vi "Self Event Alias.vi"(11 "Base Event in":refnum<class "Base Event.lvclass">) -> (2 "Self Event Alias":string)   [LabVIEW 2021, in "jettl.lvlib" / "Base Event.lvlib" / "Base Event.lvclass"]
uses:
  Base Event.lvclass
  Base Event.lvclass/Base Event.ctl
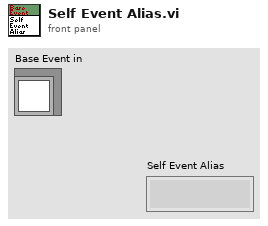
[diagram p1: front panel]
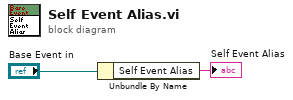
[diagram p0: block diagram]
diagram:
  n1 = Unbundle By Name("Base Event in") -> ("Self Event Alias"=→"Self Event Alias":string)
